vi "Teleop.vi"(10 "Match Info":T1={"Autonomous Elapsed Seconds"=0.0, "TeleOp Elapsed Seconds"=0.0, "Disabled Elapsed Seconds"=0.0, "Visited Autonomous"=FALSE, "Visited TeleOp"=FALSE, "Visited Disabled"=FALSE, "Autonomous Settings"={"Autonomous Style"=enum."Independent", "VI Refnum"=refnum}}, 11 "Call Context":T2) -> ()   [LabVIEW 2016]
doc: "This VI is called for each TeleOp packet received from the DS where the robot is not disabled. It is often used to read from the joysticks and update I/O or to update setpoints for timed control loops. It should complete and return within 20 milliseconds or it may miss DS packets."
uses:
  <vilib>/Rock Robotics/WPI/DriverStation/WPI_DriverStationDerivedRobotMode.ctl
  <vilib>/Rock Robotics/WPI/DriverStation/WPI_DriverStationMatch Info.ctl
  <vilib>/Rock Robotics/Network Tables/NT Read Boolean.vi
  <vilib>/Rock Robotics/Network Tables/NT Read Number.vi
  <vilib>/Rock Robotics/WPI/Utilities/WPI_GetSetVariantRefNum.vi
  <vilib>/Rock Robotics/Network Tables/NT Write Numeric Array.vi
  <vilib>/Rock Robotics/Network Tables/NT Write Boolean Array.vi
panel:
  out "Test2":dbl
  out "Test1":dbl
  out "Test Button 2":dbl
  out "Test Button 1":dbl
  out "Lift Bottom":dbl
  out "Lift Top":dbl
  out "Sample Slider 0":dbl(slide) scale=0.0..5.0
  out "Sample Boolean 1":bool
  out "Sample Boolean 0":bool
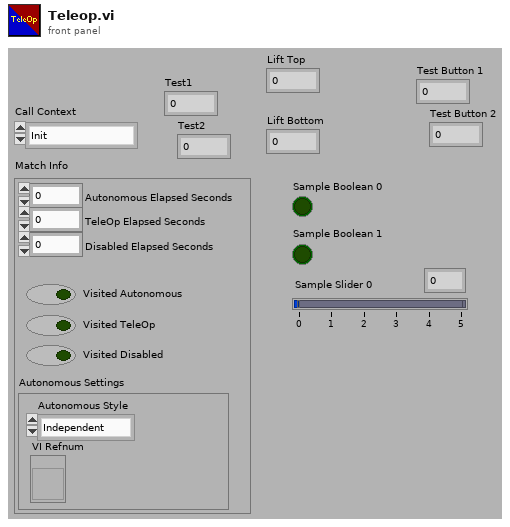
[diagram p1: front panel]
types:
  T1 = typedef "WPI_DriverStationMatch Info.ctl" = cluster{"Autonomous Elapsed Seconds":dbl, "TeleOp Elapsed Seconds":dbl, "Disabled Elapsed Seconds":dbl, "Visited Autonomous":bool, "Visited TeleOp":bool, "Visited Disabled":bool, "Autonomous Settings":cluster{"Autonomous Style":enum16{"Iterative", "Independent"}, "VI Refnum":refnum<vi>}}
  T2 = typedef "WPI_DriverStationDerivedRobotMode.ctl" = enum16{"Init", "Execute", "Stop"}
  T3 = typedef "WPI_MotorControlDeviceRef.ctl" = cluster{"DeviceStatus":errorcluster, "Type":T4, "PWM":cluster{"PWM Channel":T5, "DeadBand":T6}, "CAN":cluster{"Device Number":u8, "SetOutput VI Ref":variant, "GetOutput VI Ref":variant, "Enable VI Ref":variant, "Disable VI Ref":variant, "Data":variant}, "Invert":bool}
  T4 = typedef "WPI_MotorControlType.ctl" = enum16{"PWM", "CAN"}
  T5 = typedef "FPGA_DIOPWMChannel.ctl" = enum8{"PWM 0", "PWM 1", "PWM 2", "PWM 3", "PWM 4", "PWM 5", "PWM 6", "PWM 7", "PWM 8", "PWM 9", "PWM MXP 0", "PWM MXP 1", "PWM MXP 2", "PWM MXP 3", "PWM MXP 4", "PWM MXP 5", "PWM MXP 6", "PWM MXP 7", "PWM MXP 8", "PWM MXP 9", "Invalid"}
  T6 = typedef "WPI_PWMDeadband.ctl" = cluster{"Name":string, "maxPositivePwm":i32, "minPositivePwm":i32, "centerPwm":i32, "maxNegativePwm":i32, "minNegativePwm":i32, "angularRange":u16}
  T7 = typedef "WPI_JoystickDevRef.ctl" = cluster{"Device":T8}
  T8 = typedef "WPI_JoystickDeviceEnum.ctl" = enum16{"USB 0", "USB 1", "USB 2", "USB 3", "USB 4", "USB 5"}
  T9 = cluster{"Axes[0]":dbl, "Axes[1]":dbl, "Axes[2]":dbl, "Axes[3]":dbl, "Axes[4]":dbl, "Axes[5]":dbl, "Axes[6]":dbl, "Axes[7]":dbl, "Axes[8]":dbl}
  T10 = cluster{"Buttons[0]":bool, "Buttons[1]":bool, "Buttons[2]":bool, "Buttons[3]":bool, "Buttons[4]":bool, "Buttons[5]":bool, "Buttons[6]":bool, "Buttons[7]":bool, "Buttons[8]":bool}
  T11 = typedef "WPI_DigitalInputDevRef.ctl" = cluster{"DevStatus":errorcluster, "DIO Channel":T12}
  T12 = typedef "FPGA_DIOChannel.ctl" = enum8{"DIO 0", "DIO 1", "DIO 2", "DIO 3", "DIO 4", "DIO 5", "DIO 6", "DIO 7", "DIO 8", "DIO 9", "DIO MXP 0", "DIO MXP 1", "DIO MXP 2", "DIO MXP 3", "DIO MXP 4", "DIO MXP 5", "DIO MXP 6", "DIO MXP 7", "DIO MXP 8", "DIO MXP 9", "DIO MXP 10", "DIO MXP 11", "DIO MXP 12", "DIO MXP 13", "DIO MXP 14", "DIO MXP 15", "SPI Port CS1", "SPI Port CS2", "SPI Port CS3", "SPI Port MISO", "SPI Port MOSI", "Invalid"}
  T13 = typedef "WPI_RobotDriveDevRef.ctl" = cluster{"DevStatus":errorcluster, "Motors[]":T3[], "Square Inputs":bool, "Max Output":dbl}
  T14 = typedef "WPI_ServoDeviceRef.ctl" = cluster{"DeviceStatus":errorcluster, "PWM Channel":T5, "DeadBand":T6}
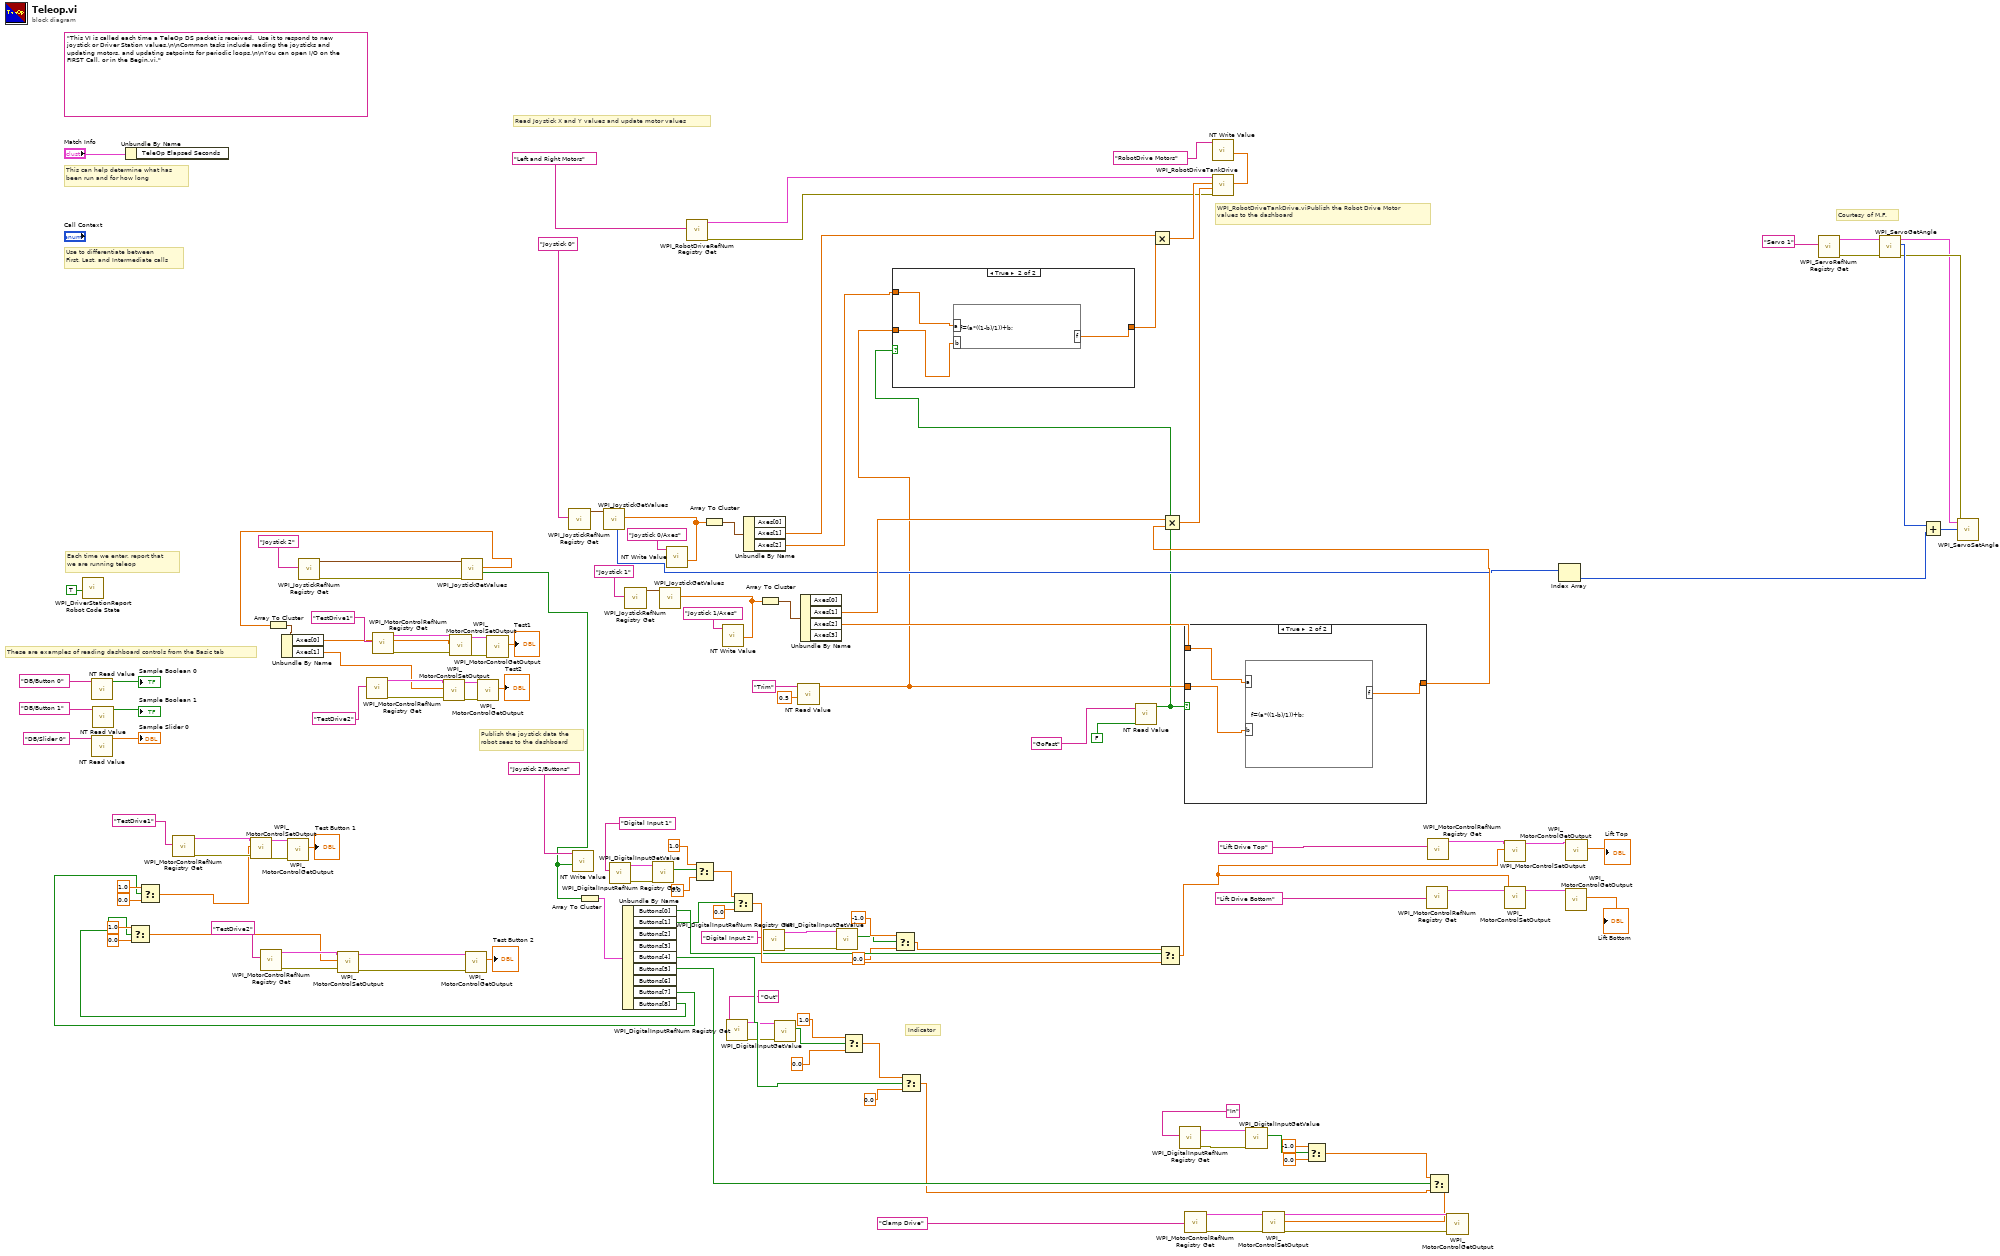
[diagram p0: block diagram]
diagram:
  (unwired) "This VI is called each time a TeleOp DS packet is received.  Use it to respond to new joystick or Driver Station values.\n\nCommon tasks include reading the joysticks and updating motors, and updating setpoints for periodic loops.\n\nYou can open I/O on the FIRST Call, or in the Begin.vi."
  # "Courtesy of M.F."
  # "Indicator"
  # "WPI_RobotDriveTankDrive.viPublish the Robot Drive Motor\nvalues to the dashboard"
  # "Publish the joystick data the\nrobot sees to the dashboard"
  # "Read Joystick X and Y values and update motor values"
  # "These are examples of reading dashboard controls from the Basic tab"
  # "Each time we enter, report that\nwe are running teleop"
  # "Use to differentiate between\nFirst, Last, and Intermediate calls"
  # "This can help determine what has\nbeen run and for how long"
  n1 = call <vilib>:"WPI_DriverStationReport Robot Code State.vi"("TeleOp"=TRUE ("Autonomous")) -> ()  [unwired: 10 in, 1 out]
  n2 = call-poly <vilib>:"NT Read Value.vi"("Name"="DB/Button 0" ("refnum name")) -> ("Boolean"=→"Sample Boolean 0":bool)  [unwired: 9 in, 1 out]
  n3 = call-poly <vilib>:"NT Read Value.vi"("Name"="DB/Slider 0" ("refnum name")) -> ("Numeric"=→"Sample Slider 0":dbl)  [unwired: 9 in, 1 out]
  n4 = call-poly <vilib>:"NT Read Value.vi"("Name"="DB/Button 1" ("refnum name")) -> ("Boolean"=→"Sample Boolean 1":bool)  [unwired: 9 in, 1 out]
  n5 = Unbundle By Name("Match Info") -> ()  [unwired: 1 out]
  n6 = call <vilib>:"WPI_MotorControlRefNum Registry Get.vi"("refnum name"="TestDrive1") -> ("error out"=w43:errorcluster, "MotorControlDevRef"=w50:T3)  [unwired: 9 in]
  n7 = call <vilib>:"WPI_MotorControlRefNum Registry Get.vi"("refnum name"="TestDrive2") -> ("error out"=w42:errorcluster, "MotorControlDevRef"=w47:T3)  [unwired: 9 in]
  n8 = call <vilib>:"WPI_JoystickRefNum Registry Get.vi"("refnum name"="Joystick 2") -> ("error out"=w51:errorcluster, "JoystickDevRef"=w95:T7)  [unwired: 9 in]
  n9 = call <vilib>:"WPI_MotorControlRefNum Registry Get.vi"("refnum name"="TestDrive2") -> ("error out"=w22:errorcluster, "MotorControlDevRef"=w27:T3)  [unwired: 9 in]
  n10 = call <vilib>:"WPI_MotorControlRefNum Registry Get.vi"("refnum name"="TestDrive1") -> ("error out"=w23:errorcluster, "MotorControlDevRef"=w30:T3)  [unwired: 9 in]
  n11 = call <vilib>:"WPI_JoystickGetValues.vi"("error in (no error)"=w51, "JoystickDevRef"=w95) -> ("Buttons"=w94:bool[], "Axes"=w18:dbl[])  [unwired: 5 in, 3 out]
  n12 = Array To Cluster(array=w18) -> (cluster=w17:T9)
  n13 = Unbundle By Name(w17) -> ("Axes[0]"=w16:dbl, "Axes[1]"=w15:dbl)
  n14 = call <vilib>:"WPI_MotorControlSetOutput.vi"("error in (no error)"=w22, "Output"=w15, "MotorControlDevRef"=w27) -> ("error out"=w19:errorcluster, "MotorControlDevRef"=w24:T3)  [unwired: 6 in, 1 out]
  n15 = call <vilib>:"WPI_MotorControlSetOutput.vi"("error in (no error)"=w23, "Output"=w16, "MotorControlDevRef"=w30) -> ("error out"=w21:errorcluster, "MotorControlDevRef"=w26:T3)  [unwired: 6 in, 1 out]
  n16 = call <vilib>:"WPI_MotorControlGetOutput.vi"("error in"=w19, "MotorControlDevRef"=w24) -> ("Output"=→"Test2":dbl)  [unwired: 7 in, 2 out]
  n17 = call <vilib>:"WPI_MotorControlGetOutput.vi"("error in"=w21, "MotorControlDevRef"=w26) -> ("Output"=→"Test1":dbl)  [unwired: 7 in, 2 out]
  n18 = call <vilib>:"WPI_JoystickRefNum Registry Get.vi"("refnum name"="Joystick 0") -> ("JoystickDevRef"=w129:T7)  [unwired: 1 in, 9 out]
  n19 = call-poly <vilib>:"NT Write Value.vi"("Boolean Array"=w94, "Name"="Joystick 2/Buttons") -> ()  [unwired: 9 in, 1 out]
  n20 = Array To Cluster(array=w94) -> (cluster=w105:T10)
  n21 = call <vilib>:"WPI_JoystickGetValues.vi"("JoystickDevRef"=w129) -> ("Axes"=w104:dbl[], "POVs"=w6:i16[])  [unwired: 6 in, 3 out]
  n22 = call <vilib>:"WPI_DigitalInputRefNum Registry Get.vi"("refnum name"="Digital Input 1") -> ("error out"=w76:errorcluster, "DigitalInputDevRef"=w77:T11)  [unwired: 9 in]
  n23 = Unbundle By Name(w105) -> ("Buttons[0]"=w96:bool, "Buttons[1]"=w73:bool, "Buttons[4]"=w70:bool, "Buttons[5]"=w72:bool, "Buttons[7]"=w32:bool, "Buttons[8]"=w31:bool)  [unwired: 3 out]
  n24 = Select(t=1.0, s=w31, f=0.0) -> (s? t:f=w36:dbl)
  n25 = Select(t=1.0, s=w32, f=0.0) -> (s? t:f=w35:dbl)
  n26 = call <vilib>:"WPI_MotorControlSetOutput.vi"("error in (no error)"=w43, "Output"=w35, "MotorControlDevRef"=w50) -> ("error out"=w41:errorcluster, "MotorControlDevRef"=w46:T3)  [unwired: 6 in, 1 out]
  n27 = call <vilib>:"WPI_MotorControlGetOutput.vi"("error in"=w41, "MotorControlDevRef"=w46) -> ("Output"=→"Test Button 1":dbl)  [unwired: 7 in, 2 out]
  n28 = call <vilib>:"WPI_MotorControlSetOutput.vi"("error in (no error)"=w42, "Output"=w36, "MotorControlDevRef"=w47) -> ("error out"=w39:errorcluster, "MotorControlDevRef"=w44:T3)  [unwired: 6 in, 1 out]
  n29 = call <vilib>:"WPI_MotorControlGetOutput.vi"("error in"=w39, "MotorControlDevRef"=w44) -> ("Output"=→"Test Button 2":dbl)  [unwired: 7 in, 2 out]
  n30 = call <vilib>:"WPI_JoystickRefNum Registry Get.vi"("refnum name"="Joystick 1") -> ("JoystickDevRef"=w10:T7)  [unwired: 1 in, 9 out]
  n31 = call <vilib>:"WPI_DigitalInputGetValue.vi"("error in (no error)"=w76, "DigitalInputDevRef"=w77) -> ("Value"=w75:bool)  [unwired: 7 in, 2 out]
  n32 = call <vilib>:"WPI_JoystickGetValues.vi"("JoystickDevRef"=w10) -> ("Axes"=w9:dbl[])  [unwired: 6 in, 4 out]
  n33 = call-poly <vilib>:"NT Write Value.vi"("Numeric Array"=w104, "Name"="Joystick 0/Axes") -> ()  [unwired: 9 in, 1 out]
  n34 = call <vilib>:"WPI_RobotDriveRefNum Registry Get.vi"("refnum name"="Left and Right Motors") -> ("error out"=w102:errorcluster, "RobotDriveDevRef"=w130:T13)  [unwired: 1 in, 8 out]
  n35 = Select(t=1.0, s=w75, f=0.0) -> (s? t:f=w86:dbl)
  n36 = Array To Cluster(array=w104) -> (cluster=w103:T9)
  n37 = call-poly <vilib>:"NT Write Value.vi"("Numeric Array"=w9, "Name"="Joystick 1/Axes") -> ()  [unwired: 9 in, 1 out]
  n38 = call <vilib>:"WPI_DigitalInputRefNum Registry Get.vi"("refnum name"="Out") -> ("error out"=w60:errorcluster, "DigitalInputDevRef"=w69:T11)  [unwired: 9 in]
  n39 = Select(t=w86, s=w73, f=0.0) -> (s? t:f=w111:dbl)
  n40 = Unbundle By Name(w103) -> ("Axes[1]"=w14:dbl, "Axes[2]"=w1:dbl)  [unwired: 1 out]
  n41 = Array To Cluster(array=w9) -> (cluster=w13:T9)
  n42 = call <vilib>:"WPI_DigitalInputRefNum Registry Get.vi"("refnum name"="Digital Input 2") -> ("error out"=w80:errorcluster, "DigitalInputDevRef"=w81:T11)  [unwired: 9 in]
  n43 = call <vilib>:"WPI_DigitalInputGetValue.vi"("error in (no error)"=w60, "DigitalInputDevRef"=w69) -> ("Value"=w67:bool)  [unwired: 7 in, 2 out]
  n44 = call-poly <vilib>:"NT Read Value.vi"("Default Value"=0.5, "Name"="Trim" ("refnum name")) -> ("Numeric"=w3:dbl)  [unwired: 8 in, 1 out]
  n45 = Unbundle By Name(w13) -> ("Axes[1]"=w8:dbl, "Axes[2]"=w7:dbl)  [unwired: 2 out]
  n46 = call <vilib>:"WPI_DigitalInputGetValue.vi"("error in (no error)"=w80, "DigitalInputDevRef"=w81) -> ("Value"=w79:bool)  [unwired: 7 in, 2 out]
  n47 = Select(t=1.0, s=w67, f=0.0) -> (s? t:f=w64:dbl)
  n48 = Select(t=-1.0, s=w79, f=0.0) -> (s? t:f=w87:dbl)
  n49 = Select(t=w64, s=w70, f=0.0) -> (s? t:f=w61:dbl)
  n50 = call-poly <vilib>:"NT Read Value.vi"("Default Value"=FALSE, "Name"="GoFast" ("refnum name")) -> ("Boolean"=w2:bool)  [unwired: 8 in, 1 out]
  n51 = case shown="True" w2 {
    tunnel: [w140 w141] -> w4
    tunnel: w3 -> [w140 w142]
    tunnel: w1 -> [_ w143]
    frame False {
    }
    frame True {
      n52 = formula code="f=(a*((1-b)/1))+b;"("a"=w143, "b"=w142) -> ("f"=w141:dbl)
    }
  }
  n53 = Multiply(x=w14, y=w4) -> (x*y=w122:dbl)
  n54 = Select(t=w87, s=w96, f=w111) -> (s? t:f=w112:dbl)
  n55 = call <vilib>:"WPI_DigitalInputRefNum Registry Get.vi"("refnum name"="In") -> ("error out"=w91:errorcluster, "DigitalInputDevRef"=w93:T11)  [unwired: 9 in]
  n56 = case shown="True" w2 {
    tunnel: [w144 w145] -> w98
    tunnel: w3 -> [w144 w146]
    tunnel: w7 -> [_ w147]
    frame False {
    }
    frame True {
      n57 = formula code="f=(a*((1-b)/1))+b;"("a"=w147, "b"=w146) -> ("f"=w145:dbl)
    }
  }
  n58 = Multiply(x=w8, y=w98) -> (x*y=w121:dbl)
  n59 = call <vilib>:"WPI_MotorControlRefNum Registry Get.vi"("refnum name"="Clamp Drive") -> ("error out"=w110:errorcluster, "MotorControlDevRef"=w108:T3)  [unwired: 9 in]
  n60 = call <vilib>:"WPI_RobotDriveTankDrive.vi"("error in (no error)"=w102, "Right axis value"=w121, "Left axis value"=w122, "RobotDriveDevRef"=w130) -> ("Motor Values"=w125:dbl[])  [unwired: 5 in, 2 out]
  n61 = call-poly <vilib>:"NT Write Value.vi"("Numeric Array"=w125, "Name"="RobotDrive Motors") -> ()  [unwired: 9 in, 1 out]
  n62 = call <vilib>:"WPI_DigitalInputGetValue.vi"("error in (no error)"=w91, "DigitalInputDevRef"=w93) -> ("Value"=w89:bool)  [unwired: 7 in, 2 out]
  n63 = Select(t=-1.0, s=w89, f=0.0) -> (s? t:f=w62:dbl)
  n64 = call <vilib>:"WPI_MotorControlRefNum Registry Get.vi"("refnum name"="Lift Drive Bottom") -> ("MotorControlDevRef"=w117:T3)  [unwired: 9 in, 1 out]
  n65 = call <vilib>:"WPI_MotorControlRefNum Registry Get.vi"("refnum name"="Lift Drive Top") -> ("MotorControlDevRef"=w118:T3)  [unwired: 9 in, 1 out]
  n66 = Select(t=w62, s=w72, f=w61) -> (s? t:f=w88:dbl)
  n67 = call <vilib>:"WPI_MotorControlSetOutput.vi"("error in (no error)"=w110, "Output"=w88, "MotorControlDevRef"=w108) -> ("error out"=w107:errorcluster, "MotorControlDevRef"=w109:T3)  [unwired: 6 in, 1 out]
  n68 = call <vilib>:"WPI_MotorControlGetOutput.vi"("error in"=w107, "MotorControlDevRef"=w109) -> ()  [unwired: 7 in, 3 out]
  n69 = call <vilib>:"WPI_MotorControlSetOutput.vi"("Output"=w112, "MotorControlDevRef"=w118) -> ("MotorControlDevRef"=w119:T3)  [unwired: 7 in, 2 out]
  n70 = call <vilib>:"WPI_MotorControlSetOutput.vi"("Output"=w112, "MotorControlDevRef"=w117) -> ("MotorControlDevRef"=w120:T3)  [unwired: 7 in, 2 out]
  n71 = Index Array(array=w6) -> (element=w5:i16)  [unwired: 1 in]
  n72 = call <vilib>:"WPI_MotorControlGetOutput.vi"("MotorControlDevRef"=w120) -> ("Output"=→"Lift Bottom":dbl)  [unwired: 8 in, 2 out]
  n73 = call <vilib>:"WPI_MotorControlGetOutput.vi"("MotorControlDevRef"=w119) -> ("Output"=→"Lift Top":dbl)  [unwired: 8 in, 2 out]
  n74 = call <vilib>:"WPI_ServoRefNum Registry Get.vi"("refnum name"="Servo 1") -> ("error out"=w55:errorcluster, "ServoDeviceRef"=w56:T14)  [unwired: 9 in]
  n75 = call <vilib>:"WPI_ServoGetAngle.vi"("ServoDeviceRef"=w56, "error in (no error)"=w55) -> ("ServoDeviceRef"=w53:T14, "Angle"=w58:u16, "error out"=w54:errorcluster)  [unwired: 6 in]
  n76 = Add(x=w58, y=w5) -> (x+y=w59:u16)
  n77 = call <vilib>:"WPI_ServoSetAngle.vi"("error in (no error)"=w54, "Angle"=w59, "ServoDeviceRef"=w53) -> ()  [unwired: 7 in, 2 out]
